vi "Add ECU Event RTM.vi"(8 "error in (no error)":errorcluster, 11 "Node Ptr":u64 format="%.0x") -> (0 "error out":errorcluster)   [LabVIEW 2011, in "Engine Sim System Explorer.lvlib"]
uses:
  Engine Sim System Explorer.lvlib
  TypeDefs/ECUEventComp.ctl
  <vilib>/NI Veristand/Custom Device API/Custom Device Channel.ctl
  <vilib>/NI Veristand/Custom Device API/Custom Device Channel Type.ctl
  Shared/Engine Simulation Global.vi
  <vilib>/NI Veristand/Custom Device API/Get Item Property (Variant).vi
  <vilib>/NI Veristand/Custom Device API/Custom Device API.lvlib
  Engine Simulation Shared.lvlib
  <vilib>/NI Veristand/Custom Device Tools/Custom Device Utility Library/Custom Device Utility Library.lvlib
panel:
  in  "Tag":string
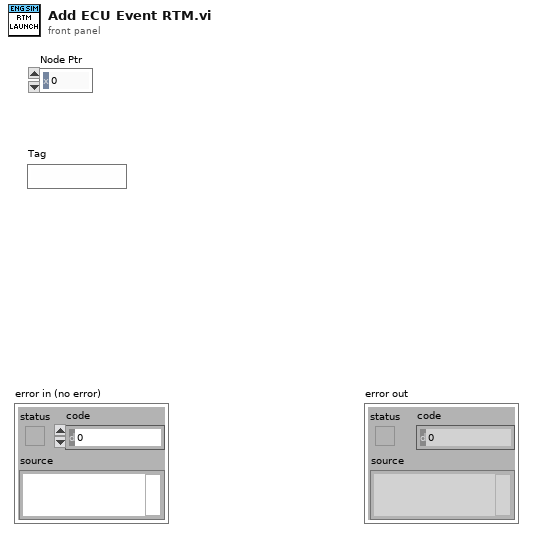
[diagram p1: front panel]
types:
  T1 = typedef "Custom Device API.lvlib/Custom Device Channel.ctl" = cluster{"Type":T2, "Units":string, "Default Value":dbl, "Faultable":bool, "Scalable":bool}
  T2 = typedef "Custom Device API.lvlib/Custom Device Channel Type.ctl" = enum16{"Input", "Output"}
  T3 = typedef "Engine Sim System Explorer.lvlib/ECUEventComp.ctl" = cluster{"Name":string, "Time Duration":bool, "Start Angle":bool, "End Angle":bool, "Angle Duration":bool}
  T4 = typedef "Custom Device API.lvlib/Custom Device Item Ref.ctl" = u64
  T5 = typedef "Custom Device API.lvlib/Custom Device Item Info.ctl" = cluster{"Name":string, "Is Channel":bool, "GUID":string}
  T6 = cluster{"Time Duration":bool, "Start Angle":bool, "End Angle":bool, "Angle Duration":bool}
  T7 = cluster{"Time Duration":bool, "Start Angle":bool, "End Angle":bool, "Angle Duration":bool}[]
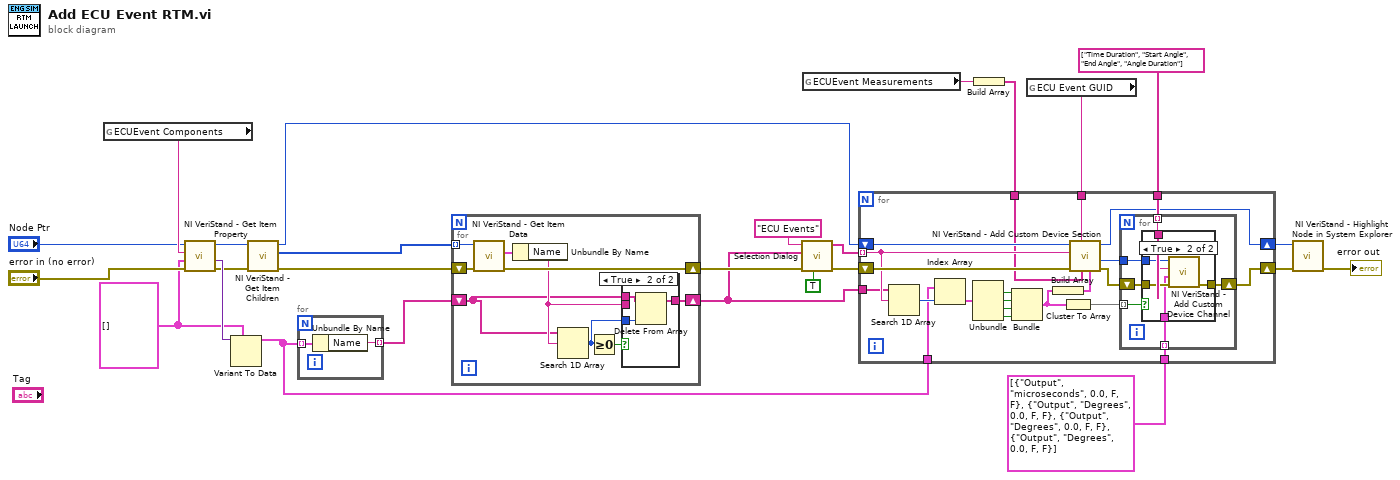
[diagram p0: block diagram]
diagram:
  w15 = T3[] [] ("ECUEvent Components")
  n1 = global read "Engine Simulation Global.vi" "ECUEvent Components"() -> (w19:string)
  n2 = call-poly <vilib>:"NI VeriStand - Get Item Property.vi"("error in (no error)"="error in (no error)", "Default Value"=w15, "Property Name"=w19, "Item Ref in"="Node Ptr") -> ("error out"=w13:errorcluster, "Value"=w16:variant, "Item Ref out"=w14:T4)  [unwired: 4 in, 1 out]
  n3 = Variant To Data(type=w15, Variant=w16) -> (data=w10:T3[])  [unwired: 1 in, 1 out]
  n4 = call <vilib>:"NI VeriStand - Get Item Children.vi"("error in (no error)"=w13, "Item Ref in"=w14) -> ("error out"=w5:errorcluster, "Child Refs"=w1:T4[], "Item Ref out"=w12:T4)  [unwired: 6 in, 1 out]
  n5 = for {
    tunnel: w10 -> [w28] mode=indexing
    tunnel: [w27] -> w3 mode=indexing
    n6 = Unbundle By Name(w28) -> ("Name"=w27:string)
  }
  n7 = for {
    shift-right: [w36] -> w4
    shift-left: w5 -> [w35]
    shift-right: [w33] -> w2
    shift-left: w3 -> [w31]
    tunnel: w1 -> [w29] mode=indexing
    n8 = call <vilib>:"NI VeriStand - Get Item Data.vi"("error in (no error)"=w35, "Item Ref in"=w29) -> ("error out"=w36:errorcluster, "Item Info"=w37:T5)  [unwired: 6 in, 2 out]
    n9 = Unbundle By Name(w37) -> ("Name"=w32:string)
    n10 = Search 1D Array(1D array=w31, element=w32) -> (index of element=w30:i32)  [unwired: 1 in]
    n11 = Greater Or Equal To 0?(x=w30) -> (x >= 0?=w34:bool)
    n12 = case shown="True" w34 {
      tunnel: [w38 w40] -> w33
      tunnel: w32 -> [_ _]
      tunnel: w31 -> [w38 w41]
      tunnel: w30 -> [_ w39]
      frame False {
      }
      frame True {
        n13 = Delete From Array(array=w41, index=w39) -> (array with subset deleted=w40:string[])  [unwired: 1 in, 1 out]
      }
    }
  }
  n14 = call "Selection Dialog.vi"("Multi-Selection?"=TRUE, "error in (no error)"=w4, "Tree Items"=w2, "Root Tag"="ECU Events") -> ("error out"=w21:errorcluster, "Selected Names"=w22:string[])  [unwired: 5 in, 1 out]
  n15 = global read "Engine Simulation Global.vi" "ECUEvent Measurements"() -> (w9:string)
  n16 = Build Array(w9) -> (w8:string[])
  n17 = global read "Engine Simulation Global.vi" "ECU Event GUID"() -> (w23:string)
  n18 = for {
    shift-right: [w43] -> w25
    shift-left: w21 -> [w62]
    shift-right: [w42] -> w26
    shift-left: w12 -> [w63]
    tunnel: w22 -> [w60] mode=indexing
    tunnel: w23 -> [w61]
    tunnel: w2 -> [w59]
    tunnel: w10 -> [w57]
    tunnel: w8 -> [w50]
    tunnel: string[] ["Time Duration", "Start Angle", "End Angle", "Angle Duration"] -> [w48]
    tunnel: T1[] [{"Type"=enum."Output", "Units"="microseconds", "Default Value"=0.0, "Faultable"=FALSE, "Scalable"=FALSE}, {"Type"=enum."Output", "Units"="Degrees", "Default Value"=0.0, "Faultable"=FALSE, "Scalable"=FALSE}, {"Type"=enum."Output", "Units"="Degrees", "Default Value"=0.0, "Faultable"=FALSE, "Scalable"=FALSE}, {"Type"=enum."Output", "Units"="Degrees", "Default Value"=0.0, "Faultable"=FALSE, "Scalable"=FALSE}] -> [w47]
    n19 = Search 1D Array(1D array=w59, element=w60) -> (index of element=w58:i32)  [unwired: 1 in]
    n20 = Index Array(array=w57, index=w58) -> (element=w56:T3)
    n21 = Unbundle(w56) -> ("Time Duration"=w55:bool, "Start Angle"=w52:bool, "End Angle"=w53:bool, "Angle Duration"=w54:bool)  [unwired: 1 out]
    n22 = Bundle("Time Duration"=w55, "Start Angle"=w52, "End Angle"=w53, "Angle Duration"=w54) -> (w46:T6)  [unwired: 1 in]
    n23 = Build Array(w46) -> (w51:T7)
    n24 = Cluster To Array(cluster=w46) -> (array=w45:bool[])
    n25 = call <vilib>:"NI VeriStand - Add Custom Device Section.vi"("Property Values"=w51, "Property names"=w50, "GUID (Default Section)"=w61, "error in (no error)"=w62, "Section Name"=w60, "Parent Ref in"=w63) -> ("error out"=w49:errorcluster, "Section Ptr"=w44:T4, "Parent Ref out"=w42:T4)  [unwired: 2 in, 1 out]
    n26 = for {
      tunnel: w44 -> [w68]
      shift-right: [w64] -> w43
      shift-left: w49 -> [w69]
      tunnel: w45 -> [w67] mode=indexing
      tunnel: w48 -> [w66] mode=indexing
      tunnel: w47 -> [w65] mode=indexing
      n27 = case shown="True" w67 {
        tunnel: w69 -> [w70 w75]
        tunnel: w68 -> [_ w74]
        tunnel: w66 -> [_ w73]
        tunnel: w65 -> [_ w72]
        tunnel: [w70 w71] -> w64
        frame False {
        }
        frame True {
          n28 = call <vilib>:"NI VeriStand - Add Custom Device Channel.vi"("error in (no error)"=w75, "Channel"=w72, "Channel Name"=w73, "Parent Ref in"=w74) -> ("error out"=w71:errorcluster)  [unwired: 4 in, 3 out]
        }
      }
    }
  }
  n29 = call <vilib>:"NI VeriStand - Highlight Node in System Explorer.vi"("error in (no error)"=w25, "Item Ref in"=w26) -> ("error out"=→"error out":errorcluster)  [unwired: 8 in, 1 out]
